vi "email message.vi"(9 "Variable Clusters":T1, 10 "Project Info":T2, 11 "User Information":T3 {"Country" items=["Afghanistan", "Aland Islands", "Albania", "Algeria", "American Samoa", "Andorra", "Angola", "Anguilla", "Antarctica", "Antigua And Barbuda", "Argentina", "Armenia", "Aruba", "Australia", "Austria", "Azerbaijan", "Bahamas", "Bahrain", "Bangladesh", "Barbados", "Belarus", "Belgium", "Belize", "Benin", "Bermuda", "Bhutan", "Bolivia", "Bosnia And Herzegovina", "Botswana", "Bouvet Island", "Brazil", "British Indian Ocean Territory", "Brunei Darussalam", "Bulgaria", "Burkina Faso", "Burundi", "Cambodia", "Cameroon", "Canada", "Cape Verde", "Cayman Islands", "Central African Republic", "Chad", "Chile", "China", "Christmas Island", "Cocos (Keeling) Islands", "Colombia", "Comoros", "Congo", "Congo, The Democratic Republic Of The", "Cook Islands", "Costa Rica", "Cote D'Ivoire", "Croatia", "Cuba", "Cyprus", "Czech Republic", "Denmark", "Djibouti", "Dominica", "Dominican Republic", "Ecuador", "Egypt", "El Salvador", "Equatorial Guinea", "Eritrea", "Estonia", "Ethiopia", "Falkland Islands (Malvinas)", "Faroe Islands", "Fiji", "Finland", "France", "French Guiana", "French Polynesia", "French Southern Territories", "Gabon", "Gambia", "Georgia", "Germany", "Ghana", "Gibraltar", "Greece", "Greenland", "Grenada", "Guadeloupe", "Guam", "Guatemala", "Guernsey", "Guinea", "Guinea-Bissau", "Guyana", "Haiti", "Heard Island And Mcdonald Islands", "Holy See (Vatican City State)", "Honduras", "Hong Kong", "Hungary", "Iceland", "India", "Indonesia", "Iran, Islamic Republic Of", "Iraq", "Ireland", "Isle Of Man", "Israel", "Italy", "Jamaica", "Japan", "Jersey", "Jordan", "Kazakhstan", "Kenya", "Kiribati", "Korea, Democratic People'S Republic Of", "Korea, Republic Of", "Kuwait", "Kyrgyzstan", "Lao People'S Democratic Republic", "Latvia", "Lebanon", "Lesotho", "Liberia", "Libyan Arab Jamahiriya", "Liechtenstein", "Lithuania", "Luxembourg", "Macao", "Macedonia, The Former Yugoslav Republic Of", "Madagascar", "Malawi", "Malaysia", "Maldives", "Mali", "Malta", "Marshall Islands", "Martinique", "Mauritania", "Mauritius", "Mayotte", "Mexico", "Micronesia, Federated States Of", "Moldova, Republic Of", "Monaco", "Mongolia", "Montserrat", "Morocco", "Mozambique", "Myanmar", "Namibia", "Nauru", "Nepal", "Netherlands", "Netherlands Antilles", "New Caledonia", "New Zealand", "Nicaragua", "Niger", "Nigeria", "Niue", "Norfolk Island", "Northern Mariana Islands", "Norway", "Oman", "Pakistan", "Palau", "Palestinian Territory, Occupied", "Panama", "Papua New Guinea", "Paraguay", "Peru", "Philippines", "Pitcairn", "Poland", "Portugal", "Puerto Rico", "Qatar", "Reunion", "Romania", "Russian Federation", "Rwanda", "Saint Helena", "Saint Kitts And Nevis", "Saint Lucia", "Saint Pierre And Miquelon", "Saint Vincent And The Grenadines", "Samoa", "San Marino", "Sao Tome And Principe", "Saudi Arabia", "Senegal", "Serbia And Montenegro", "Seychelles", "Sierra Leone", "Singapore", "Slovakia", "Slovenia", "Solomon Islands", "Somalia", "South Africa", "South Georgia And The South Sandwich Islands", "Spain", "Sri Lanka", "Sudan", "Suriname", "Svalbard And Jan Mayen", "Swaziland", "Sweden", "Switzerland", "Syrian Arab Republic", "Taiwan, Province Of China", "Tajikistan", "Tanzania, United Republic Of", "Thailand", "Timor-Leste", "Togo", "Tokelau", "Tonga", "Trinidad And Tobago", "Tunisia", "Turkey", "Turkmenistan", "Turks And Caicos Islands", "Tuvalu", "Uganda", "Ukraine", "United Arab Emirates", "United Kingdom", "United States", "United States Minor Outlying Islands", "Uruguay", "Uzbekistan", "Vanuatu", "Venezuela", "Viet Nam", "Virgin Islands, British", "Virgin Islands, U.S.", "Wallis And Futuna", "Western Sahara", "Yemen", "Zambia", "Zimbabwe", "(Not Specified)"]}) -> (3 "Message":string)   [LabVIEW 2015]
uses:
  User Information.ctl
  Country Ring.ctl
  Project inputs.ctl
  Variable cluster.ctl
  AguaClara Library.lvlib
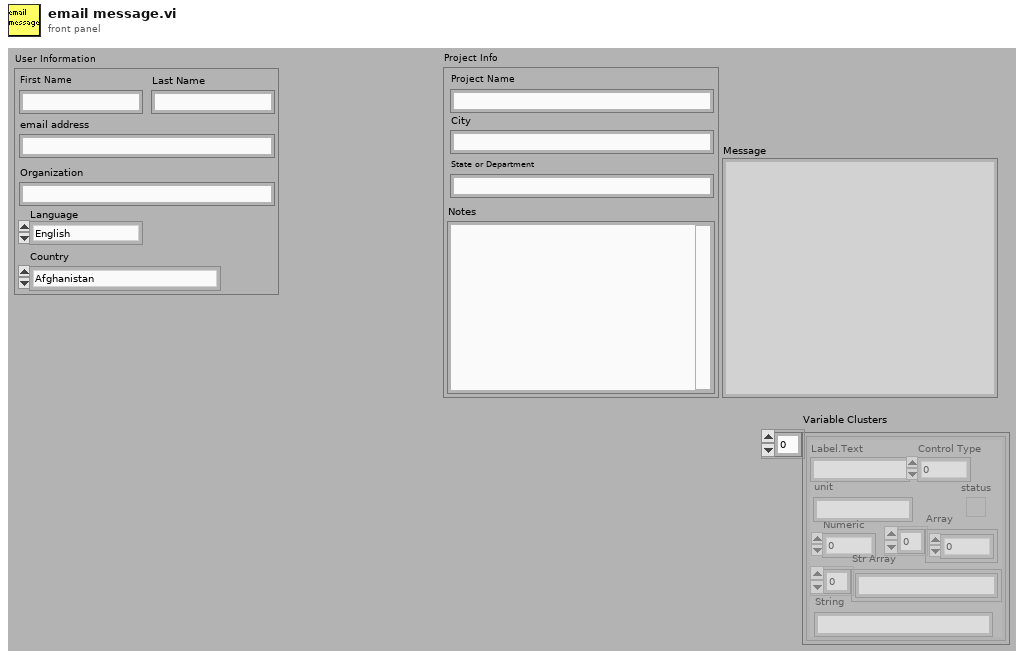
[diagram p1: front panel]
types:
  T1 = typedef "Variable cluster.ctl" = cluster{"Label.Text":string, "Control Type":u32, "Numeric":dbl, "Array":dbl[], "status":bool, "Str Array":string[], "String":string, "unit":string}[]
  T2 = typedef "AguaClara Library.lvlib/Project inputs.ctl" = cluster{"Project Name":string, "City":string, "State":string, "Notes":string}
  T3 = typedef "AguaClara Library.lvlib/User Information.ctl" = cluster{"First Name":string, "Last Name":string, "Email Address":string, "Organization":string, "Language":enum16{"English", "Español", "French"}, "Country":T4}
  T4 = typedef "Country Ring.ctl" = u16
  T5 = cluster{"Label.Text":string, "Control Type":u32, "Numeric":dbl, "Array":dbl[], "status":bool, "Str Array":string[], "String":string, "unit":string}
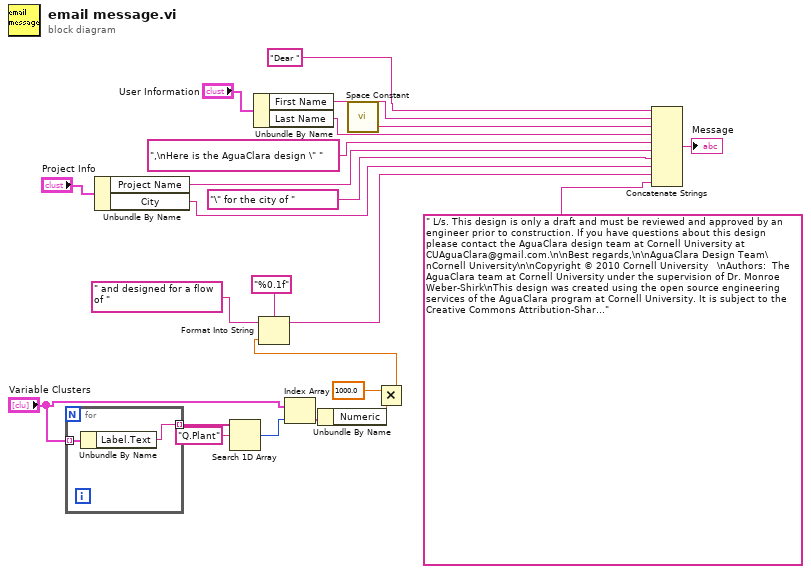
[diagram p0: block diagram]
diagram:
  n1 = for {
    tunnel: "Variable Clusters" -> [w25] mode=indexing
    tunnel: [w24] -> w8 mode=indexing
    n2 = Unbundle By Name(w25) -> ("Label.Text"=w24:string)
  }
  n3 = Unbundle By Name("Project Info") -> ("Project Name"=w16:string, "City"=w14:string)
  n4 = Search 1D Array(1D array=w8, element="Q.Plant") -> (index of element=w5:i32)  [unwired: 1 in]
  n5 = Unbundle By Name("User Information") -> ("First Name"=w21:string, "Last Name"=w19:string)
  n6 = Index Array(array="Variable Clusters", index=w5) -> (element=w4:T5)
  n7 = Unbundle By Name(w4) -> ("Numeric"=w3:dbl)
  n8 = call <vilib>:"Space Constant.vi"() -> ("String"=w20:string)
  n9 = Multiply(x=1000.0, y=w3) -> (x*y=w2:dbl)
  n10 = Format Into String(format string="%0.1f", initial string=" and designed for a flow of ", w2) -> (resulting string=w13:string)  [unwired: 1 in, 1 out]
  n11 = Concatenate Strings("Dear ", w21, w20, w19, ",\nHere is the AguaClara design \" ", w16, "\" for the city of ", w14, w13, " L/s. This design is only a draft and must be reviewed and approved by an engineer prior to construction. If you have questions about this design please contact the AguaClara design team at Cornell University at CUAguaClara@gmail.com.\n\nBest regards,\n\nAguaClara Design Team\nCornell University\n\nCopyright © 2010 Cornell University   \nAuthors:  The AguaClara team at Cornell University under the supervision of Dr. Monroe Weber-Shirk\nThis design was created using the open source engineering services of the AguaClara program at Cornell University. It is subject to the Creative Commons Attribution-ShareAlike 3.0 United States license. If you alter, transform, or build upon this work, you may distribute the resulting work only under the same, similar or a compatible license.\nPermission to use this AguaClara Design Tool along with the subsequent AutoCAD renderings and supporting files for design specifications provided by Cornell based on your input parameters (collectively \"WORK\") and their associated copyrights without a written agreement is hereby granted. Any water treatment plants built using this WORK shall be designed and supervised by a licensed civil engineer.\nIN NO EVENT SHALL CCTEC, CORNELL UNIVERSITY, OR THEIR EMPLOYEES BE LIABLE TO ANY PARTY FOR DIRECT, INDIRECT, SPECIAL, INCIDENTAL, OR CONSEQUENTIAL DAMAGES, INCLUDING LOST PROFITS, ARISING OUT OF THE USE OF WORK AND ITS ASSOCIATED COPYRIGHTS, EVEN IF CCTEC OR CORNELL MAY HAVE BEEN ADVISED OF THE POSSIBILITY OF SUCH DAMAGE.\nTHE WORK PROVIDED HEREIN IS ON AN \"AS IS\" BASIS, AND CCTEC, CORNELL, AND THEIR EMPLOYEES HAVE NO OBLIGATION TO PROVIDE MAINTENANCE, SUPPORT, UPDATES, ENHANCEMENTS, OR MODIFICATIONS.  CCTEC, CORNELL, AND THEIR EMPLOYEES MAKE NO REPRESENTATIONS AND EXTEND NO WARRANTIES OF ANY KIND, EITHER IMPLIED OR EXPRESSED, INCLUDING, BUT NOT LIMITED TO, THE IMPLIED WARRANTIES OF MERCHANTABILITY OR FITNESS FOR A PARTICULAR PURPOSE, OR THAT THE USE OF WORK AND ITS ASSOCIATED COPYRIGHTS WILL NOT INFRINGE ANY PATENT, TRADEMARK OR OTHER RIGHTS.\nUsers of WORK shall indemnify, hold harmless and defend Cornell, its officers, employees, agents, and the sponsors of the research that let to WORK against any and all claims, suits, losses, damage, costs, fees, and expenses resulting from or arising out of use of WORK.  This indemnification shall include, but not be limited to, any product liability.  Users of WORK, at their sole cost and expense, shall sufficiently insure their activities in connection with the WORK and obtain, keep in force, and maintain insurance or an equivalent program of self insurance.  Cornell shall notify users of WORK in writing of any claim or suit brought against Cornell in respect of which Cornell intends to invoke the provisions of this paragraph.  Users of WORK shall keep Cornell informed on a current basis of its defense of any claims under this paragraph.  ") -> (→"Message":string)
